vi "Global_var.vi"() -> ()   [LabVIEW 2012]
panel:
  out "base-path":path=path "C:/Users/mclmcgill/Desktop/Stroke_Perceptual_Testing"
  in  "Visual Ctrl?":bool
  in  "Zref":dbl
  in  "Yref":dbl
  in  "Xref":dbl
  in  "Total_trial":u8=50 max=40 step=5
  out "Curl value":i8=10
  out "Damping":i16=8
  out "Stiffness":i16=1800
  in  "Movement dist.":u8=15 max=40 step=5
  out "Center_XYZ":dbl[](array[numeric])
  out "Min.direction":i8
  out "Language":bool
  out "Last Name":string
  out "First Name":string
  # "Reference position for minimum jerk/hold"
  # "Stiffness value\ncan be changed \nand set as default"
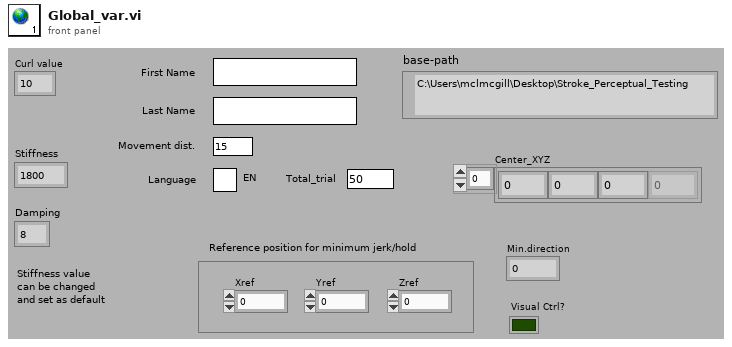
[diagram p1: front panel]
diagram:
